vi "example_02_convert.vi"() -> ()   [LabVIEW 2015, in "lv-unit-conversion.lvlib"] (continued)
in", "name"="thirty-second of inch", "dimension"="L", "is_si_unit"=TRUE, "category"="derived", "base_unit"="m", "conversion_reference"="DERIVED", "is_exact"=TRUE, "a"=0.0, "b"=0.0254, "c"=32.0, "d"=0.0, "underlying_def"="", "description"=""}, {"symbol"="1/64 in", "name"="sixty-fourth of inch", "dimension"="L", "is_si_unit"=TRUE, "category"="derived", "base_unit"="m", "conversion_reference"="DERIVED", "is_exact"=TRUE, "a"=0.0, "b"=0.0254, "c"=64.0, "d"=0.0, "underlying_def"="", "description"=""}, {"symbol"="10 ft", "name"="ten foot", "dimension"="L", "is_si_unit"=TRUE, "category"="derived", "base_unit"="m", "conversion_reference"="DERIVED", "is_exact"=TRUE, "a"=0.0, "b"=3.048, "c"=1.0, "d"=0.0, "underlying_def"="", "description"=""}, {"symbol"="10 in", "name"="ten inch", "dimension"="L", "is_si_unit"=TRUE, "category"="derived", "base_unit"="m", "conversion_reference"="DERIVED", "is_exact"=TRUE, "a"=0.0, "b"=0.254, "c"=1.0, "d"=0.0, "underlying_def"="", "description"=""}, {"symbol"="10 km", "name"="10 kilometre", "dimension"="L", "is_si_unit"=TRUE, "category"="derived", "base_unit"="m", "conversion_reference"="DERIVED", "is_exact"=TRUE, "a"=0.0, "b"=10000.0, "c"=1.0, "d"=0.0, "underlying_def"="", "description"=""}, {"symbol"="100 ft", "name"="hundred foot", "dimension"="L", "is_si_unit"=TRUE, "category"="derived", "base_unit"="m", "conversion_reference"="DERIVED", "is_exact"=TRUE, "a"=0.0, "b"=30.48, "c"=1.0, "d"=0.0, "underlying_def"="", "description"=""}, {"symbol"="100 km", "name"="100 kilometre", "dimension"="L", "is_si_unit"=TRUE, "category"="derived", "base_unit"="m", "conversion_reference"="DERIVED", "is_exact"=TRUE, "a"=0.0, "b"=100000.0, "c"=1.0, "d"=0.0, "underlying_def"="", "description"=""}, {"symbol"="1000 ft", "name"="thousand foot", "dimension"="L", "is_si_unit"=TRUE, "category"="derived", "base_unit"="m", "conversion_reference"="DERIVED", "is_exact"=TRUE, "a"=0.0, "b"=304.8, "c"=1.0, "d"=0.0, "underlying_def"="", "description"=""}, {"symbol"="30 ft", "name"="thirty foot", "dimension"="L", "is_si_unit"=TRUE, "category"="derived", "base_unit"="m", "conversion_reference"="DERIVED", "is_exact"=TRUE, "a"=0.0, "b"=9.144, "c"=1.0, "d"=0.0, "underlying_def"="", "description"=""}, {"symbol"="30 m", "name"="thirty metres", "dimension"="L", "is_si_unit"=TRUE, "category"="derived", "base_unit"="m", "conversion_reference"="DERIVED", "is_exact"=TRUE, "a"=0.0, "b"=30.0, "c"=1.0, "d"=0.0, "underlying_def"="", "description"=""}, {"symbol"="1E6 bbl/acre", "name"="million barrel per acre", "dimension"="L", "is_si_unit"=TRUE, "category"="derived", "base_unit"="m3/m2", "conversion_reference"="DERIVED", "is_exact"=TRUE, "a"=0.0, "b"=2464298142777.8574, "c"=62726400000.0, "d"=0.0, "underlying_def"="", "description"=""}, {"symbol"="bbl/acre", "name"="barrel per acre", "dimension"="L", "is_si_unit"=TRUE, "category"="derived", "base_unit"="m3/m2", "conversion_reference"="DERIVED", "is_exact"=TRUE, "a"=0.0, "b"=2464298.1427778574, "c"=62726400000.0, "d"=0.0, "underlying_def"="", "description"=""}, {"symbol"="ft3/ft2", "name"="cubic foot per square foot", "dimension"="L", "is_si_unit"=TRUE, "category"="derived", "base_unit"="m3/m2", "conversion_reference"="DERIVED", "is_exact"=TRUE, "a"=0.0, "b"=0.3048, "c"=1.0, "d"=0.0, "underlying_def"="", "description"=""}, {"symbol"="cm", "name"="centimetre", "dimension"="L", "is_si_unit"=TRUE, "category"="prefixed", "base_unit"="m", "conversion_reference"="DERIVED", "is_exact"=TRUE, "a"=0.0, "b"=0.01, "c"=1.0, "d"=0.0, "underlying_def"="", "description"=""}, {"symbol"="dam", "name"="dekametre", "dimension"="L", "is_si_unit"=TRUE, "category"="prefixed", "base_unit"="m", "conversion_reference"="DERIVED", "is_exact"=TRUE, "a"=0.0, "b"=10.0, "c"=1.0, "d"=0.0, "underlying_def"="", "description"=""}, {"symbol"="dm", "name"="decimetre", "dimension"="L", "is_si_unit"=TRUE, "category"="prefixed", "base_unit"="m", "conversion_reference"="DERIVED", "is_exact"=TRUE, "a"=0.0, "b"=0.1, "c"=1.0, "d"=0.0, "underlying_def"="", "description"=""}, {"symbol"="Em", "name"="exametre", "dimension"="L", "is_si_unit"=TRUE, "category"="prefixed", "base_unit"="m", "conversion_reference"="DERIVED", "is_exact"=TRUE, "a"=0.0, "b"=1e+18, "c"=1.0, "d"=0.0, "underlying_def"="", "description"=""}, {"symbol"="fm", "name"="femtometre", "dimension"="L", "is_si_unit"=TRUE, "category"="prefixed", "base_unit"="m", "conversion_reference"="DERIVED", "is_exact"=TRUE, "a"=0.0, "b"=1e-15, "c"=1.0, "d"=0.0, "underlying_def"="", "description"=""}, {"symbol"="Gm", "name"="gigametre", "dimension"="L", "is_si_unit"=TRUE, "category"="prefixed", "base_unit"="m", "conversion_reference"="DERIVED", "is_exact"=TRUE, "a"=0.0, "b"=1000000000.0, "c"=1.0, "d"=0.0, "underlying_def"="", "description"=""}, {"symbol"="hm", "name"="hectometre", "dimension"="L", "is_si_unit"=TRUE, "category"="prefixed", "base_unit"="m", "conversion_reference"="DERIVED", "is_exact"=TRUE, "a"=0.0, "b"=100.0, "c"=1.0, "d"=0.0, "underlying_def"="", "description"=""}, {"symbol"="km", "name"="kilometre", "dimension"="L", "is_si_unit"=TRUE, "category"="prefixed", "base_unit"="m", "conversion_reference"="DERIVED", "is_exact"=TRUE, "a"=0.0, "b"=1000.0, "c"=1.0, "d"=0.0, "underlying_def"="", "description"=""}, {"symbol"="Mm", "name"="megametre", "dimension"="L", "is_si_unit"=TRUE, "category"="prefixed", "base_unit"="m", "conversion_reference"="DERIVED", "is_exact"=TRUE, "a"=0.0, "b"=1000000.0, "c"=1.0, "d"=0.0, "underlying_def"="", "description"=""}, {"symbol"="mm", "name"="millimetre", "dimension"="L", "is_si_unit"=TRUE, "category"="prefixed", "base_unit"="m", "conversion_reference"="DERIVED", "is_exact"=TRUE, "a"=0.0, "b"=0.001, "c"=1.0, "d"=0.0, "underlying_def"="", "description"=""}, {"symbol"="nm", "name"="nanometre", "dimension"="L", "is_si_unit"=TRUE, "category"="prefixed", "base_unit"="m", "conversion_reference"="DERIVED", "is_exact"=TRUE, "a"=0.0, "b"=1e-09, "c"=1.0, "d"=0.0, "underlying_def"="", "description"=""}, {"symbol"="pm", "name"="picometre", "dimension"="L", "is_si_unit"=TRUE, "category"="prefixed", "base_unit"="m", "conversion_reference"="DERIVED", "is_exact"=TRUE, "a"=0.0, "b"=1e-12, "c"=1.0, "d"=0.0, "underlying_def"="", "description"=""}, {"symbol"="Tm", "name"="terametre", "dimension"="L", "is_si_unit"=TRUE, "category"="prefixed", "base_unit"="m", "conversion_reference"="DERIVED", "is_exact"=TRUE, "a"=0.0, "b"=1000000000000.0, "c"=1.0, "d"=0.0, "underlying_def"="", "description"=""}, {"symbol"="um", "name"="micrometre", "dimension"="L", "is_si_unit"=TRUE, "category"="prefixed", "base_unit"="m", "conversion_reference"="DERIVED", "is_exact"=TRUE, "a"=0.0, "b"=1e-06, "c"=1.0, "d"=0.0, "underlying_def"="", "description"="Sometimes called a micron."}, {"symbol"="m/deltaK", "name"="metre per delta kelvin", "dimension"="L/D", "is_si_unit"=TRUE, "category"="derived", "base_unit"="", "conversion_reference"="", "is_exact"=FALSE, "a"=0.0, "b"=0.0, "c"=0.0, "d"=0.0, "underlying_def"="", "description"=""}, {"symbol"="ft/deltaF", "name"="foot per delta Fahrenheit", "dimension"="L/D", "is_si_unit"=TRUE, "category"="derived", "base_unit"="m/deltaK", "conversion_reference"="DERIVED", "is_exact"=TRUE, "a"=0.0, "b"=2.7432, "c"=5.0, "d"=0.0, "underlying_def"="", "description"=""}, {"symbol"="m/kg", "name"="metre per kilogram", "dimension"="L/M", "is_si_unit"=TRUE, "category"="derived", "base_unit"="", "conversion_reference"="", "is_exact"=FALSE, "a"=0.0, "b"=0.0, "c"=0.0, "d"=0.0, "underlying_def"="", "description"=""}, {"symbol"="ft/lbm", "name"="foot per pound-mass", "dimension"="L/M", "is_si_unit"=TRUE, "category"="derived", "base_unit"="m/kg", "conversion_reference"="DERIVED", "is_exact"=TRUE, "a"=0.0, "b"=0.3048, "c"=0.45359237, "d"=0.0, "underlying_def"="", "description"=""}, {"symbol"="knot", "name"="knot", "dimension"="L/T", "is_si_unit"=TRUE, "category"="atom-allowed", "base_unit"="m/s", "conversion_reference"="NIST-SI", "is_exact"=TRUE, "a"=0.0, "b"=1852.0, "c"=3600.0, "d"=0.0, "underlying_def"="mi[naut]/h", "description"="The knot is defined as one nautical mile per hour."}, {"symbol"="m/s", "name"="metre per second", "dimension"="L/T", "is_si_unit"=TRUE, "category"="derived", "base_unit"="", "conversion_reference"="", "is_exact"=FALSE, "a"=0.0, "b"=0.0, "c"=0.0, "d"=0.0, "underlying_def"="", "description"=""}, {"symbol"="m3/(s.m2)", "name"="cubic metre per second square metre", "dimension"="L/T", "is_si_unit"=TRUE, "category"="derived", "base_unit"="", "conversion_reference"="", "is_exact"=FALSE, "a"=0.0, "b"=0.0, "c"=0.0, "d"=0.0, "underlying_def"="m/s", "description"=""}, {"symbol"="1000 ft/h", "name"="thousand foot per hour", "dimension"="L/T", "is_si_unit"=TRUE, "category"="derived", "base_unit"="m/s", "conversion_reference"="DERIVED", "is_exact"=TRUE, "a"=0.0, "b"=304.8, "c"=3600.0, "d"=0.0, "underlying_def"="", "description"=""}, {"symbol"="1000 ft/s", "name"="thousand foot per second", "dimension"="L/T", "is_si_unit"=TRUE, "category"="derived", "base_unit"="m/s", "conversion_reference"="DERIVED", "is_exact"=TRUE, "a"=0.0, "b"=304.8, "c"=1.0, "d"=0.0, "underlying_def"="", "description"=""}, {"symbol"="cm/a", "name"="centimetre per julian-year", "dimension"="L/T", "is_si_unit"=TRUE, "category"="derived", "base_unit"="m/s", "conversion_reference"="DERIVED", "is_exact"=TRUE, "a"=0.0, "b"=0.01, "c"=31557600.0, "d"=0.0, "underlying_def"="", "description"=""}, {"symbol"="cm/s", "name"="centimetre per second", "dimension"="L/T", "is_si_unit"=TRUE, "category"="derived", "base_unit"="m/s", "conversion_reference"="DERIVED", "is_exact"=TRUE, "a"=0.0, "b"=0.01, "c"=1.0, "d"=0.0, "underlying_def"="", "description"=""}, {"symbol"="dm/s", "name"="decimetre per second", "dimension"="L/T", "is_si_unit"=TRUE, "category"="derived", "base_unit"="m/s", "conversion_reference"="DERIVED", "is_exact"=TRUE, "a"=0.0, "b"=0.1, "c"=1.0, "d"=0.0, "underlying_def"="", "description"=""}, {"symbol"="ft/d", "name"="foot per day", "dimension"="L/T", "is_si_unit"=TRUE, "category"="derived", "base_unit"="m/s", "conversion_reference"="DERIVED", "is_exact"=TRUE, "a"=0.0, "b"=0.3048, "c"=86400.0, "d"=0.0, "underlying_def"="", "description"=""}, {"symbol"="ft/h", "name"="foot per hour", "dimension"="L/T", "is_si_unit"=TRUE, "category"="derived", "base_unit"="m/s", "conversion_reference"="DERIVED", "is_exact"=TRUE, "a"=0.0, "b"=0.3048, "c"=3600.0, "d"=0.0, "underlying_def"="", "description"=""}, {"symbol"="ft/min", "name"="foot per minute", "dimension"="L/T", "is_si_unit"=TRUE, "category"="derived", "base_unit"="m/s", "conversion_reference"="DERIVED", "is_exact"=TRUE, "a"=0.0, "b"=0.3048, "c"=60.0, "d"=0.0, "underlying_def"="", "description"=""}, {"symbol"="ft/ms", "name"="foot per millisecond", "dimension"="L/T", "is_si_unit"=TRUE, "category"="derived", "base_unit"="m/s", "conversion_reference"="DERIVED", "is_exact"=TRUE, "a"=0.0, "b"=304.8, "c"=1.0, "d"=0.0, "underlying_def"="", "description"=""}, {"symbol"="ft/s", "name"="foot per second", "dimension"="L/T", "is_si_unit"=TRUE, "category"="derived", "base_unit"="m/s", "conversion_reference"="DERIVED", "is_exact"=TRUE, "a"=0.0, "b"=0.3048, "c"=1.0, "d"=0.0, "underlying_def"="", "description"=""}, {"symbol"="ft/us", "name"="foot per microsecond", "dimension"="L/T", "is_si_unit"=TRUE, "category"="derived", "base_unit"="m/s", "conversion_reference"="DERIVED", "is_exact"=TRUE, "a"=0.0, "b"=304800.0, "c"=1.0, "d"=0.0, "underlying_def"="", "description"=""}, {"symbol"="in/a", "name"="inch per julian-year", "dimension"="L/T", "is_si_unit"=TRUE, "category"="derived", "base_unit"="m/s", "conversion_reference"="DERIVED", "is_exact"=TRUE, "a"=0.0, "b"=0.0254, "c"=31557600.0, "d"=0.0, "underlying_def"="", "description"=""}, {"symbol"="in/min", "name"="inch per minute", "dimension"="L/T", "is_si_unit"=TRUE, "category"="derived", "base_unit"="m/s", "conversion_reference"="DERIVED", "is_exact"=TRUE, "a"=0.0, "b"=0.0254, "c"=60.0, "d"=0.0, "underlying_def"="", "description"=""}, {"symbol"="in/s", "name"="inch per second", "dimension"="L/T", "is_si_unit"=TRUE, "category"="derived", "base_unit"="m/s", "conversion_reference"="DERIVED", "is_exact"=TRUE, "a"=0.0, "b"=0.0254, "c"=1.0, "d"=0.0, "underlying_def"="", "description"=""}, {"symbol"="km/h", "name"="kilometre per hour", "dimension"="L/T", "is_si_unit"=TRUE, "category"="derived", "base_unit"="m/s", "conversion_reference"="DERIVED", "is_exact"=TRUE, "a"=0.0, "b"=1.0, "c"=3.6, "d"=0.0, "underlying_def"="", "description"=""}, {"symbol"="km/s", "name"="kilometre per second", "dimension"="L/T", "is_si_unit"=TRUE, "category"="derived", "base_unit"="m/s", "conversion_reference"="DERIVED", "is_exact"=TRUE, "a"=0.0, "b"=1000.0, "c"=1.0, "d"=0.0, "underlying_def"="", "description"=""}, {"symbol"="m/d", "name"="metre per day", "dimension"="L/T", "is_si_unit"=TRUE, "category"="derived", "base_unit"="m/s", "conversion_reference"="DERIVED", "is_exact"=TRUE, "a"=0.0, "b"=1.0, "c"=86400.0, "d"=0.0, "underlying_def"="", "description"=""}, {"symbol"="m/h", "name"="metre per hour", "dimension"="L/T", "is_si_unit"=TRUE, "category"="derived", "base_unit"="m/s", "conversion_reference"="DERIVED", "is_exact"=TRUE, "a"=0.0, "b"=1.0, "c"=3600.0, "d"=0.0, "underlying_def"="", "description"=""}, {"symbol"="m/min", "name"="metre per minute", "dimension"="L/T", "is_si_unit"=TRUE, "category"="derived", "base_unit"="m/s", "conversion_reference"="DERIVED", "is_exact"=TRUE, "a"=0.0, "b"=1.0, "c"=60.0, "d"=0.0, "underlying_def"="", "description"=""}, {"symbol"="m/ms", "name"="metre per millisecond", "dimension"="L/T", "is_si_unit"=TRUE, "category"="derived", "base_unit"="m/s", "conversion_reference"="DERIVED", "is_exact"=TRUE, "a"=0.0, "b"=1000.0, "c"=1.0, "d"=0.0, "underlying_def"="", "description"=""}, {"symbol"="mi/h", "name"="mile per hour", "dimension"="L/T", "is_si_unit"=TRUE, "category"="derived", "base_unit"="m/s", "conversion_reference"="DERIVED", "is_exact"=TRUE, "a"=0.0, "b"=1609.344, "c"=3600.0, "d"=0.0, "underlying_def"="", "description"=""}, {"symbol"="mil/a", "name"="mil per julian-year", "dimension"="L/T", "is_si_unit"=TRUE, "category"="derived", "base_unit"="m/s", "conversion_reference"="DERIVED", "is_exact"=TRUE, "a"=0.0, "b"=2.54e-05, "c"=31557600.0, "d"=0.0, "underlying_def"="", "description"=""}, {"symbol"="mm/a", "name"="millimetre per julian-year", "dimension"="L/T", "is_si_unit"=TRUE, "category"="derived", "base_unit"="m/s", "conversion_reference"="DERIVED", "is_exact"=TRUE, "a"=0.0, "b"=0.001, "c"=31557600.0, "d"=0.0, "underlying_def"="", "description"=""}, {"symbol"="mm/s", "name"="millimetre per second", "dimension"="L/T", "is_si_unit"=TRUE, "category"="derived", "base_unit"="m/s", "conversion_reference"="DERIVED", "is_exact"=TRUE, "a"=0.0, "b"=0.001, "c"=1.0, "d"=0.0, "underlying_def"="", "description"=""}, {"symbol"="nm/s", "name"="nanometre per second", "dimension"="L/T", "is_si_unit"=TRUE, "category"="derived", "base_unit"="m/s", "conversion_reference"="DERIVED", "is_exact"=TRUE, "a"=0.0, "b"=1e-09, "c"=1.0, "d"=0.0, "underlying_def"="", "description"=""}, {"symbol"="um/s", "name"="micrometre per second", "dimension"="L/T", "is_si_unit"=TRUE, "category"="derived", "base_unit"="m/s", "conversion_reference"="DERIVED", "is_exact"=TRUE, "a"=0.0, "b"=1e-06, "c"=1.0, "d"=0.0, "underlying_def"="", "description"=""}, {"symbol"="ft3/(min.ft2)", "name"="cubic foot per minute square foot", "dimension"="L/T", "is_si_unit"=TRUE, "category"="derived", "base_unit"="m3/(s.m2)", "conversion_reference"="DERIVED", "is_exact"=TRUE, "a"=0.0, "b"=0.3048, "c"=60.0, "d"=0.0, "underlying_def"="", "description"=""}, {"symbol"="ft3/(s.ft2)", "name"="cubic foot per second square foot", "dimension"="L/T", "is_si_unit"=TRUE, "category"="derived", "base_unit"="m3/(s.m2)", "conversion_reference"="DERIVED", "is_exact"=TRUE, "a"=0.0, "b"=0.3048, "c"=1.0, "d"=0.0, "underlying_def"="", "description"=""}, {"symbol"="gal[UK]/(h.ft2)", "name"="UK gallon per hour square foot", "dimension"="L/T", "is_si_unit"=TRUE, "category"="derived", "base_unit"="m3/(s.m2)", "conversion_reference"="DERIVED", "is_exact"=TRUE, "a"=0.0, "b"=0.00454609, "c"=334.450944, "d"=0.0, "underlying_def"="", "description"=""}, {"symbol"="gal[UK]/(h.in2)", "name"="UK gallon per hour square inch", "dimension"="L/T", "is_si_unit"=TRUE, "category"="derived", "base_unit"="m3/(s.m2)", "conversion_reference"="DERIVED", "is_exact"=TRUE, "a"=0.0, "b"=0.00454609, "c"=2.322576, "d"=0.0, "underlying_def"="", "description"=""}, {"symbol"="gal[UK]/(min.ft2)", "name"="UK gallon per minute square foot", "dimension"="L/T", "is_si_unit"=TRUE, "category"="derived", "base_unit"="m3/(s.m2)", "conversion_reference"="DERIVED", "is_exact"=TRUE, "a"=0.0, "b"=0.00454609, "c"=5.5741824, "d"=0.0, "underlying_def"="", "description"=""}, {"symbol"="gal[US]/(h.ft2)", "name"="US gallon per hour square foot", "dimension"="L/T", "is_si_unit"=TRUE, "category"="derived", "base_unit"="m3/(s.m2)", "conversion_reference"="DERIVED", "is_exact"=TRUE, "a"=0.0, "b"=0.003785411784, "c"=334.450944, "d"=0.0, "underlying_def"="", "description"=""}, {"symbol"="gal[US]/(h.in2)", "name"="US gallon per hour square inch", "dimension"="L/T", "is_si_unit"=TRUE, "category"="derived", "base_unit"="m3/(s.m2)", "conversion_reference"="DERIVED", "is_exact"=TRUE, "a"=0.0, "b"=0.003785411784, "c"=2.322576, "d"=0.0, "underlying_def"="", "description"=""}, {"symbol"="gal[US]/(min.ft2)", "name"="US gallon per minute square foot", "dimension"="L/T", "is_si_unit"=TRUE, "category"="derived", "base_unit"="m3/(s.m2)", "conversion_reference"="DERIVED", "is_exact"=TRUE, "a"=0.0, "b"=0.003785411784, "c"=5.5741824, "d"=0.0, "underlying_def"="", "description"=""}, {"symbol"="Gal", "name"="galileo", "dimension"="L/T2", "is_si_unit"=TRUE, "category"="atom", "base_unit"="m/s2", "conversion_reference"="NIST-SI", "is_exact"=TRUE, "a"=0.0, "b"=0.01, "c"=1.0, "d"=0.0, "underlying_def"="cm/s2", "description"="The gal is employed in geodesy and geophysics to express acceleration due to gravity."}, {"symbol"="gn", "name"="gravity", "dimension"="L/T2", "is_si_unit"=TRUE, "category"="atom", "base_unit"="m/s2", "conversion_reference"="NIST-SI", "is_exact"=TRUE, "a"=0.0, "b"=9.80665, "c"=1.0, "d"=0.0, "underlying_def"="", "description"="The standard acceleration due to gravity on Earth."}, {"symbol"="m/s2", "name"="metre per second squared", "dimension"="L/T2", "is_si_unit"=TRUE, "category"="derived", "base_unit"="", "conversion_reference"="", "is_exact"=FALSE, "a"=0.0, "b"=0.0, "c"=0.0, "d"=0.0, "underlying_def"="", "description"=""}, {"symbol"="cm/s2", "name"="centimetre per square second", "dimension"="L/T2", "is_si_unit"=TRUE, "category"="derived", "base_unit"="m/s2", "conversion_reference"="DERIVED", "is_exact"=TRUE, "a"=0.0, "b"=0.01, "c"=1.0, "d"=0.0, "underlying_def"="", "description"=""}, {"symbol"="ft/s2", "name"="foot per second squared", "dimension"="L/T2", "is_si_unit"=TRUE, "category"="derived", "base_unit"="m/s2", "conversion_reference"="DERIVED", "is_exact"=TRUE, "a"=0.0, "b"=0.3048, "c"=1.0, "d"=0.0, "underlying_def"="", "description"=""}, {"symbol"="in/s2", "name"="inch per second squared", "dimension"="L/T2", "is_si_unit"=TRUE, "category"="derived", "base_unit"="m/s2", "conversion_reference"="DERIVED", "is_exact"=TRUE, "a"=0.0, "b"=0.0254, "c"=1.0, "d"=0.0, "underlying_def"="", "description"=""}, {"symbol"="mGal", "name"="milligalileo", "dimension"="L/T2", "is_si_unit"=TRUE, "category"="prefixed", "base_unit"="m/s2", "conversion_reference"="DERIVED", "is_exact"=TRUE, "a"=0.0, "b"=1e-05, "c"=1.0, "d"=0.0, "underlying_def"="", "description"=""}, {"symbol"="mgn", "name"="thousandth of gravity", "dimension"="L/T2", "is_si_unit"=TRUE, "category"="prefixed", "base_unit"="m/s2", "conversion_reference"="DERIVED", "is_exact"=TRUE, "a"=0.0, "b"=0.00980665, "c"=1.0, "d"=0.0, "underlying_def"="", "description"=""}, {"symbol"="TD[API]", "name"="teradarcy-API", "dimension"="L2", "is_si_unit"=TRUE, "category"="atom-allowed", "base_unit"="", "conversion_reference"="", "is_exact"=FALSE, "a"=0.0, "b"=0.0, "c"=0.0, "d"=0.0, "underlying_def"="m2", "description"="The API teradarcy is numerically equal to a metre squared."}, {"symbol"="acre", "name"="acre", "dimension"="L2", "is_si_unit"=TRUE, "category"="atom", "base_unit"="m2", "conversion_reference"="NIST-44", "is_exact"=TRUE, "a"=0.0, "b"=62726400000.0, "c"=15499969.0, "d"=0.0, "underlying_def"="43560 ft[US]2", "description"="US survey acre. Equal to 43,560 square survey foot (exactly). From NIST."}, {"symbol"="b", "name"="barn", "dimension"="L2", "is_si_unit"=TRUE, "category"="atom-allowed", "base_unit"="m2", "conversion_reference"="NIST-SI", "is_exact"=TRUE, "a"=0.0, "b"=1e-28, "c"=1.0, "d"=0.0, "underlying_def"="100 fm2", "description"="The barn is a unit of area employed to express cross sections in nuclear physics."}, {"symbol"="ha", "name"="hectare", "dimension"="L2", "is_si_unit"=TRUE, "category"="atom-allowed", "base_unit"="m2", "conversion_reference"="NIST-SI", "is_exact"=TRUE, "a"=0.0, "b"=10000.0, "c"=1.0, "d"=0.0, "underlying_def"="10000 m2", "description"="Used to express agrarian area."}, {"symbol"="section", "name"="section", "dimension"="L2", "is_si_unit"=TRUE, "category"="atom", "base_unit"="m2", "conversion_reference"="NIST-44", "is_exact"=TRUE, "a"=0.0, "b"=40144896000000.0, "c"=15499969.0, "d"=0.0, "underlying_def"="640 acre", "description"="640 acres or 1 square US survey mile."}, {"symbol"="D", "name"="darcy", "dimension"="L2", "is_si_unit"=TRUE, "category"="atom", "base_unit"="TD[API]", "conversion_reference"="DEFINITION", "is_exact"=TRUE, "a"=0.0, "b"=1e-12, "c"=1.01325, "d"=0.0, "underlying_def"="", "description"="The darcy is a unit for expressing the permeability of porous solids, not area (from NIST-SI). \n\t\t\t\tOne darcy is the permeability of a solid through which one cubic centimeter of fluid, having a \n\t\t\t\tviscosity of one centipoise, will flow in one second through a section one centimeter thick and one \n\t\t\t\tsquare centimeter in cross section, if the pressure difference between the two sides of the solid is \n\t\t\t\tone atmosphere (from Russ Rowlett's \"A Dictionary of Units of Measurement\" at \n\t\t\t\thttp://www.unc.edu/~rowlett/units/). \n\t\t\t\tThus, 1 D=(1 cm3)(1 cP)/((1 s)(1 cm2)(1 atm/cm))=1 cm.cP/(atm.s/cm)=1 cm2.cP/atm.s=(1E-4 m2)(1E-3 \n\t\t\t\tPa.s)/(1.01325E5 Pa.s)=1E-12/1.01325 m2 [exactly]. \n\t\t\t\tAlso see, Wangen, Magnus (2010) Physical Principles of Sedimentary Basin Analysis (page 12), \n\t\t\t\tCambridge, UK New York: Cambridge University Press, 2010. \n\t\t\t\tISBN 978-0-511-71237-1.\n\t\t\t"}, {"symbol"="D[API]", "name"="darcy-API", "dimension"="L2", "is_si_unit"=TRUE, "category"="atom-allowed", "base_unit"="TD[API]", "conversion_reference"="API-MPMS15", "is_exact"=TRUE, "a"=0.0, "b"=1e-12, "c"=1.0, "d"=0.0, "underlying_def"="um2", "description"="The darcy is a unit of permeability in fluid flow through a porous medium, having the dimensions of \n\t\t\t\tdynamic viscosity multiplied by volume flowrate per unit area and divided by pressure gradient, \n\t\t\t\twhich simplifies to a dimension of area. \n\t\t\t\tA darcy is defined as being exactly equal to 1 um2. \n\t\t\t\tA permeability of one darcy will permit a flow of 1 m3/s of fluid of 1 Pa.s viscosity through an \n\t\t\t\tarea of 1 m2 under a pressure gradient of 10**12 Pa/m.\n\t\t\t"}, {"symbol"="m3/m", "name"="cubic metre per metre", "dimension"="L2", "is_si_unit"=TRUE, "category"="derived", "base_unit"="", "conversion_reference"="", "is_exact"=FALSE, "a"=0.0, "b"=0.0, "c"=0.0, "d"=0.0, "underlying_def"="m2", "description"=""}, {"symbol"="cm2", "name"="square centimetre", "dimension"="L2", "is_si_unit"=TRUE, "category"="derived", "base_unit"="m2", "conversion_reference"="DERIVED", "is_exact"=TRUE, "a"=0.0, "b"=0.0001, "c"=1.0, "d"=0.0, "underlying_def"="", "description"=""}, {"symbol"="km2", "name"="square kilometre", "dimension"="L2", "is_si_unit"=TRUE, "category"="derived", "base_unit"="m2", "conversion_reference"="DERIVED", "is_exact"=TRUE, "a"=0.0, "b"=1000000.0, "c"=1.0, "d"=0.0, "underlying_def"="", "description"=""}, {"symbol"="mm2", "name"="square millimetre", "dimension"="L2", "is_si_unit"=TRUE, "category"="derived", "base_unit"="m2", "conversion_reference"="DERIVED", "is_exact"=TRUE, "a"=0.0, "b"=1e-06, "c"=1.0, "d"=0.0, "underlying_def"="", "description"=""}, {"symbol"="um2", "name"="square micrometre", "dimension"="L2", "is_si_unit"=TRUE, "category"="derived", "base_unit"="m2", "conversion_reference"="DERIVED", "is_exact"=TRUE, "a"=0.0, "b"=1e-12, "c"=1.0, "d"=0.0, "underlying_def"="", "description"=""}, {"symbol"="0.01 dm3/km", "name"="cubic decimetre per hundred kilometre", "dimension"="L2", "is_si_unit"=TRUE, "category"="derived", "base_unit"="m3/m", "conversion_reference"="DERIVED", "is_exact"=TRUE, "a"=0.0, "b"=1e-08, "c"=1.0, "d"=0.0, "underlying_def"="", "description"=""}, {"symbol"="0.01 L/km", "name"="litre per hundred kilometre", "dimension"="L2", "is_si_unit"=TRUE, "category"="derived", "base_unit"="m3/m", "conversion_reference"="DERIVED", "is_exact"=TRUE, "a"=0.0, "b"=1e-08, "c"=1.0, "d"=0.0, "underlying_def"="", "description"=""}, {"symbol"="bbl/ft", "name"="barrel per foot", "dimension"="L2", "is_si_unit"=TRUE, "category"="derived", "base_unit"="m3/m", "conversion_reference"="DERIVED", "is_exact"=TRUE, "a"=0.0, "b"=0.158987294928, "c"=0.3048, "d"=0.0, "underlying_def"="", "description"=""}, {"symbol"="bbl/in", "name"="barrel per inch", "dimension"="L2", "is_si_unit"=TRUE, "category"="derived", "base_unit"="m3/m", "conversion_reference"="DERIVED", "is_exact"=TRUE, "a"=0.0, "b"=0.158987294928, "c"=0.0254, "d"=0.0, "underlying_def"="", "description"=""}, {"symbol"="bbl/mi", "name"="barrel per mile", "dimension"="L2", "is_si_unit"=TRUE, "category"="derived", "base_unit"="m3/m", "conversion_reference"="DERIVED", "is_exact"=TRUE, "a"=0.0, "b"=0.158987294928, "c"=1609.344, "d"=0.0, "underlying_def"="", "description"=""}, {"symbol"="dm3/m", "name"="cubic decimetre per metre", "dimension"="L2", "is_si_unit"=TRUE, "category"="derived", "base_unit"="m3/m", "conversion_reference"="DERIVED", "is_exact"=TRUE, "a"=0.0, "b"=0.001, "c"=1.0, "d"=0.0, "underlying_def"="", "description"=""}, {"symbol"="ft3/ft", "name"="cubic foot per foot", "dimension"="L2", "is_si_unit"=TRUE, "category"="derived", "base_unit"="m3/m", "conversion_reference"="DERIVED", "is_exact"=TRUE, "a"=0.0, "b"=0.09290304, "c"=1.0, "d"=0.0, "underlying_def"="", "description"=""}, {"symbol"="gal[UK]/mi", "name"="UK gallon per mile", "dimension"="L2", "is_si_unit"=TRUE, "category"="derived", "base_unit"="m3/m", "conversion_reference"="DERIVED", "is_exact"=TRUE, "a"=0.0, "b"=0.00454609, "c"=1609.344, "d"=0.0, "underlying_def"="", "description"=""}, {"symbol"="gal[US]/ft", "name"="US gallon per foot", "dimension"="L2", "is_si_unit"=TRUE, "category"="derived", "base_unit"="m3/m", "conversion_reference"="DERIVED", "is_exact"=TRUE, "a"=0.0, "b"=0.003785411784, "c"=0.3048, "d"=0.0, "underlying_def"="", "description"=""}, {"symbol"="gal[US]/mi", "name"="US gallon per mile", "dimension"="L2", "is_si_unit"=TRUE, "category"="derived", "base_unit"="m3/m", "conversion_reference"="DERIVED", "is_exact"=TRUE, "a"=0.0, "b"=0.003785411784, "c"=1609.344, "d"=0.0, "underlying_def"="", "description"=""}, {"symbol"="in3/ft", "name"="cubic inch per foot", "dimension"="L2", "is_si_unit"=TRUE, "category"="derived", "base_unit"="m3/m", "conversion_reference"="DERIVED", "is_exact"=TRUE, "a"=0.0, "b"=1.6387064e-05, "c"=0.3048, "d"=0.0, "underlying_def"="", "description"=""}, {"symbol"="L/m", "name"="litre per metre", "dimension"="L2", "is_si_unit"=TRUE, "category"="derived", "base_unit"="m3/m", "conversion_reference"="DERIVED", "is_exact"=TRUE, "a"=0.0, "b"=0.001, "c"=1.0, "d"=0.0, "underlying_def"="", "description"=""}, {"symbol"="m3/km", "name"="cubic metre per kilometre", "dimension"="L2", "is_si_unit"=TRUE, "category"="derived", "base_unit"="m3/m", "conversion_reference"="DERIVED", "is_exact"=TRUE, "a"=0.0, "b"=0.001, "c"=1.0, "d"=0.0, "underlying_def"="", "description"=""}, {"symbol"="m2", "name"="square metre", "dimension"="L2", "is_si_unit"=TRUE, "category"="derived", "base_unit"="", "conversion_reference"="", "is_exact"=FALSE, "a"=0.0, "b"=0.0, "c"=0.0, "d"=0.0, "underlying_def"="", "description"=""}, {"symbol"="ft2", "name"="square foot", "dimension"="L2", "is_si_unit"=TRUE, "category"="derived", "base_unit"="m2", "conversion_reference"="DERIVED", "is_exact"=TRUE, "a"=0.0, "b"=0.09290304, "c"=1.0, "d"=0.0, "underlying_def"="", "description"=""}, {"symbol"="in2", "name"="square inch", "dimension"="L2", "is_si_unit"=TRUE, "category"="derived", "base_unit"="m2", "conversion_reference"="DERIVED", "is_exact"=TRUE, "a"=0.0, "b"=0.00064516, "c"=1.0, "d"=0.0, "underlying_def"="", "description"=""}, {"symbol"="mi[US]2", "name"="square US survey mile", "dimension"="L2", "is_si_unit"=TRUE, "category"="derived", "base_unit"="m2", "conversion_reference"="DERIVED", "is_exact"=TRUE, "a"=0.0, "b"=40144896000000.0, "c"=15499969.0, "d"=0.0, "underlying_def"="", "description"=""}, {"symbol"="mi2", "name"="square mile", "dimension"="L2", "is_si_unit"=TRUE, "category"="derived", "base_unit"="m2", "conversion_reference"="DERIVED", "is_exact"=TRUE, "a"=0.0, "b"=2589988.110336, "c"=1.0, "d"=0.0, "underlying_def"="", "description"=""}, {"symbol"="yd2", "name"="square yard", "dimension"="L2", "is_si_unit"=TRUE, "category"="derived", "base_unit"="m2", "conversion_reference"="DERIVED", "is_exact"=TRUE, "a"=0.0, "b"=0.83612736, "c"=1.0, "d"=0.0, "underlying_def"="", "description"=""}, {"symbol"="mD", "name"="millidarcy", "dimension"="L2", "is_si_unit"=TRUE, "category"="prefixed", "base_unit"="TD[API]", "conversion_reference"="DERIVED", "is_exact"=TRUE, "a"=0.0, "b"=1e-15, "c"=1.01325, "d"=0.0, "underlying_def"="", "description"=""}, {"symbol"="J/(kg.deltaK)", "name"="joule per kilogram delta kelvin", "dimension"="L2/DT2", "is_si_unit"=TRUE, "category"="derived", "base_unit"="", "conversion_reference"="", "is_exact"=FALSE, "a"=0.0, "b"=0.0, "c"=0.0, "d"=0.0, "underlying_def"="", "description"=""}, {"symbol"="Btu[IT]/(lbm.deltaF)", "name"="BTU per pound-mass delta Fahrenheit", "dimension"="L2/DT2", "is_si_unit"=TRUE, "category"="derived", "base_unit"="J/(kg.deltaK)", "conversion_reference"="DERIVED", "is_exact"=TRUE, "a"=0.0, "b"=4186.8, "c"=1.0, "d"=0.0, "underlying_def"="", "description"=""}, {"symbol"="Btu[IT]/(lbm.deltaR)", "name"="BTU per pound-mass delta Rankine", "dimension"="L2/DT2", "is_si_unit"=TRUE, "category"="derived", "base_unit"="J/(kg.deltaK)", "conversion_reference"="DERIVED", "is_exact"=TRUE, "a"=0.0, "b"=4186.8, "c"=1.0, "d"=0.0, "underlying_def"="", "description"=""}, {"symbol"="cal[th]/(g.deltaK)", "name"="calorie per gram delta kelvin", "dimension"="L2/DT2", "is_si_unit"=TRUE, "category"="derived", "base_unit"="J/(kg.deltaK)", "conversion_reference"="DERIVED", "is_exact"=TRUE, "a"=0.0, "b"=4184.0, "c"=1.0, "d"=0.0, "underlying_def"="", "description"=""}, {"symbol"="J/(g.deltaK)", "name"="joule per gram delta kelvin", "dimension"="L2/DT2", "is_si_unit"=TRUE, "category"="derived", "base_unit"="J/(kg.deltaK)", "conversion_reference"="DERIVED", "is_exact"=TRUE, "a"=0.0, "b"=1000.0, "c"=1.0, "d"=0.0, "underlying_def"="", "description"=""}, {"symbol"="kcal[th]/(kg.deltaC)", "name"="thousand calorie per kilogram delta Celsius", "dimension"="L2/DT2", "is_si_unit"=TRUE, "category"="derived", "base_unit"="J/(kg.deltaK)", "conversion_reference"="DERIVED", "is_exact"=TRUE, "a"=0.0, "b"=4184.0, "c"=1.0, "d"=0.0, "underlying_def"="", "description"=""}, {"symbol"="kJ/(kg.deltaK)", "name"="kilojoule per kilogram delta kelvin", "dimension"="L2/DT2", "is_si_unit"=TRUE, "category"="derived", "base_unit"="J/(kg.deltaK)", "conversion_reference"="DERIVED", "is_exact"=TRUE, "a"=0.0, "b"=1000.0, "c"=1.0, "d"=0.0, "underlying_def"="", "description"=""}, {"symbol"="kW.h/(kg.deltaC)", "name"="kilowatt hour per kilogram delta Celsius", "dimension"="L2/DT2", "is_si_unit"=TRUE, "category"="derived", "base_unit"="J/(kg.deltaK)", "conversion_reference"="DERIVED", "is_exact"=TRUE, "a"=0.0, "b"=3600000.0, "c"=1.0, "d"=0.0, "underlying_def"="", "description"=""}, {"symbol"="m2/kg", "name"="square metre per kilogram", "dimension"="L2/M", "is_si_unit"=TRUE, "category"="derived", "base_unit"="", "conversion_reference"="", "is_exact"=FALSE, "a"=0.0, "b"=0.0, "c"=0.0, "d"=0.0, "underlying_def"="", "description"=""}, {"symbol"="cm2/g", "name"="square centimetre per gram", "dimension"="L2/M", "is_si_unit"=TRUE, "category"="derived", "base_unit"="m2/kg", "conversion_reference"="DERIVED", "is_exact"=TRUE, "a"=0.0, "b"=0.1, "c"=1.0, "d"=0.0, "underlying_def"="", "description"=""}, {"symbol"="ft2/lbm", "name"="square foot per pound-mass", "dimension"="L2/M", "is_si_unit"=TRUE, "category"="derived", "base_unit"="m2/kg", "conversion_reference"="DERIVED", "is_exact"=TRUE, "a"=0.0, "b"=0.09290304, "c"=0.45359237, "d"=0.0, "underlying_def"="", "description"=""}, {"symbol"="m2/g", "name"="square metre per gram", "dimension"="L2/M", "is_si_unit"=TRUE, "category"="derived", "base_unit"="m2/kg", "conversion_reference"="DERIVED", "is_exact"=TRUE, "a"=0.0, "b"=1000.0, "c"=1.0, "d"=0.0, "underlying_def"="", "description"=""}, {"symbol"="m2/mol", "name"="square metre per gram-mole", "dimension"="L2/N", "is_si_unit"=TRUE, "category"="derived", "base_unit"="", "conversion_reference"="", "is_exact"=FALSE, "a"=0.0, "b"=0.0, "c"=0.0, "d"=0.0, "underlying_def"="", "description"=""}, {"symbol"="St", "name"="stokes", "dimension"="L2/T", "is_si_unit"=TRUE, "category"="atom", "base_unit"="m2/s", "conversion_reference"="NIST-SI", "is_exact"=TRUE, "a"=0.0, "b"=0.0001, "c"=1.0, "d"=0.0, "underlying_def"="cm2/s", "description"="The stokes is the CGS unit for kinematic viscosity."}, {"symbol"="m2/s", "name"="square metre per second", "dimension"="L2/T", "is_si_unit"=TRUE, "category"="derived", "base_unit"="", "conversion_reference"="", "is_exact"=FALSE, "a"=0.0, "b"=0.0, "c"=0.0, "d"=0.0, "underlying_def"="", "description"=""}, {"symbol"="m3/(s.m)", "name"="cubic metre per second metre", "dimension"="L2/T", "is_si_unit"=TRUE, "category"="derived", "base_unit"="", "conversion_reference"="", "is_exact"=FALSE, "a"=0.0, "b"=0.0, "c"=0.0, "d"=0.0, "underlying_def"="m2/s", "description"=""}, {"symbol"="mol.m2/(mol.s)", "name"="mole square metre per mole second", "dimension"="L2/T", "is_si_unit"=TRUE, "category"="derived", "base_unit"="", "conversion_reference"="", "is_exact"=FALSE, "a"=0.0, "b"=0.0, "c"=0.0, "d"=0.0, "underlying_def"="m2/s", "description"=""}, {"symbol"="Pa.s.m3/kg", "name"="pascal second square metre per kilogram", "dimension"="L2/T", "is_si_unit"=TRUE, "category"="derived", "base_unit"="", "conversion_reference"="", "is_exact"=FALSE, "a"=0.0, "b"=0.0, "c"=0.0, "d"=0.0, "underlying_def"="m2/s", "description"=""}, {"symbol"="W.m2.deltaK/(J.deltaK)", "name"="watt square metre delta kelvin per joule delta kelvin", "dimension"="L2/T", "is_si_unit"=TRUE, "category"="derived", "base_unit"="", "conversion_reference"="", "is_exact"=FALSE, "a"=0.0, "b"=0.0, "c"=0.0, "d"=0.0, "underlying_def"="m2/s", "description"=""}, {"symbol"="cm2/s", "name"="square centimetre per second", "dimension"="L2/T", "is_si_unit"=TRUE, "category"="derived", "base_unit"="m2/s", "conversion_reference"="DERIVED", "is_exact"=TRUE, "a"=0.0, "b"=0.0001, "c"=1.0, "d"=0.0, "underlying_def"="", "description"=""}, {"symbol"="ft2/h", "name"="square foot per hour", "dimension"="L2/T", "is_si_unit"=TRUE, "category"="derived", "base_unit"="m2/s", "conversion_reference"="DERIVED", "is_exact"=TRUE, "a"=0.0, "b"=0.09290304, "c"=3600.0, "d"=0.0, "underlying_def"="", "description"=""}, {"symbol"="ft2/s", "name"="square foot per second", "dimension"="L2/T", "is_si_unit"=TRUE, "category"="derived", "base_unit"="m2/s", "conversion_reference"="DERIVED", "is_exact"=TRUE, "a"=0.0, "b"=0.09290304, "c"=1.0, "d"=0.0, "underlying_def"="", "description"=""}, {"symbol"="in2/s", "name"="square inch per second", "dimension"="L2/T", "is_si_unit"=TRUE, "category"="derived", "base_unit"="m2/s", "conversion_reference"="DERIVED", "is_exact"=TRUE, "a"=0.0, "b"=0.00064516, "c"=1.0, "d"=0.0, "underlying_def"="", "description"=""}, {"symbol"="m2/d", "name"="square metre per day", "dimension"="L2/T", "is_si_unit"=TRUE, "category"="derived", "base_unit"="m2/s", "conversion_reference"="DERIVED", "is_exact"=TRUE, "a"=0.0, "b"=1.0, "c"=86400.0, "d"=0.0, "underlying_def"="", "description"=""}, {"symbol"="m2/h", "name"="square metre per hour", "dimension"="L2/T", "is_si_unit"=TRUE, "category"="derived", "base_unit"="m2/s", "conversion_reference"="DERIVED", "is_exact"=TRUE, "a"=0.0, "b"=1.0, "c"=3600.0, "d"=0.0, "underlying_def"="", "description"=""}, {"symbol"="mm2/s", "name"="square millimetre per second", "dimension"="L2/T", "is_si_unit"=TRUE, "category"="derived", "base_unit"="m2/s", "conversion_reference"="DERIVED", "is_exact"=TRUE, "a"=0.0, "b"=1e-06, "c"=1.0, "d"=0.0, "underlying_def"="", "description"=""}, {"symbol"="1000 ft3/(d.ft)", "name"="(thousand cubic foot per day) per foot", "dimension"="L2/T", "is_si_unit"=TRUE, "category"="derived", "base_unit"="m3/(s.m)", "conversion_reference"="DERIVED", "is_exact"=TRUE, "a"=0.0, "b"=28.316846592, "c"=26334.72, "d"=0.0, "underlying_def"="", "description"=""}, {"symbol"="1000 m3/(d.m)", "name"="(thousand cubic metre per day) per metre", "dimension"="L2/T", "is_si_unit"=TRUE, "category"="derived", "base_unit"="m3/(s.m)", "conversion_reference"="DERIVED", "is_exact"=TRUE, "a"=0.0, "b"=1000.0, "c"=86400.0, "d"=0.0, "underlying_def"="", "description"=""}, {"symbol"="1000 m3/(h.m)", "name"="(thousand cubic metre per hour) per metre", "dimension"="L2/T", "is_si_unit"=TRUE, "category"="derived", "base_unit"="m3/(s.m)", "conversion_reference"="DERIVED", "is_exact"=TRUE, "a"=0.0, "b"=1000.0, "c"=3600.0, "d"=0.0, "underlying_def"="", "description"=""}, {"symbol"="bbl/(d.ft)", "name"="barrel per day foot", "dimension"="L2/T", "is_si_unit"=TRUE, "category"="derived", "base_unit"="m3/(s.m)", "conversion_reference"="DERIVED", "is_exact"=TRUE, "a"=0.0, "b"=0.158987294928, "c"=26334.72, "d"=0.0, "underlying_def"="", "description"=""}, {"symbol"="ft3/(d.ft)", "name"="(cubic foot per day) per foot", "dimension"="L2/T", "is_si_unit"=TRUE, "category"="derived", "base_unit"="m3/(s.m)", "conversion_reference"="DERIVED", "is_exact"=TRUE, "a"=0.0, "b"=0.09290304, "c"=86400.0, "d"=0.0, "underlying_def"="", "description"=""}, {"symbol"="gal[UK]/(h.ft)", "name"="UK gallon per hour foot", "dimension"="L2/T", "is_si_unit"=TRUE, "category"="derived", "base_unit"="m3/(s.m)", "conversion_reference"="DERIVED", "is_exact"=TRUE, "a"=0.0, "b"=0.00454609, "c"=1097.28, "d"=0.0, "underlying_def"="", "description"=""}, {"symbol"="gal[UK]/(h.in)", "name"="UK gallon per hour inch", "dimension"="L2/T", "is_si_unit"=TRUE, "category"="derived", "base_unit"="m3/(s.m)", "conversion_reference"="DERIVED", "is_exact"=TRUE, "a"=0.0, "b"=0.00454609, "c"=91.44, "d"=0.0, "underlying_def"="", "description"=""}, {"symbol"="gal[UK]/(min.ft)", "name"="UK gallon per minute foot", "dimension"="L2/T", "is_si_unit"=TRUE, "category"="derived", "base_unit"="m3/(s.m)", "conversion_reference"="DERIVED", "is_exact"=TRUE, "a"=0.0, "b"=0.00454609, "c"=18.288, "d"=0.0, "underlying_def"="", "description"=""}, {"symbol"="gal[US]/(h.ft)", "name"="US gallon per hour foot", "dimension"="L2/T", "is_si_unit"=TRUE, "category"="derived", "base_unit"="m3/(s.m)", "conversion_reference"="DERIVED", "is_exact"=TRUE, "a"=0.0, "b"=0.003785411784, "c"=1097.28, "d"=0.0, "underlying_def"="", "description"=""}, {"symbol"="gal[US]/(h.in)", "name"="US gallon per hour inch", "dimension"="L2/T", "is_si_unit"=TRUE, "category"="derived", "base_unit"="m3/(s.m)", "conversion_reference"="DERIVED", "is_exact"=TRUE, "a"=0.0, "b"=0.003785411784, "c"=91.44, "d"=0.0, "underlying_def"="", "description"=""}, {"symbol"="gal[US]/(min.ft)", "name"="US
